vi "Process BD Preview.vi"(9 "Visible Area":T2, 11 "vi ref in":refnum<vi>) -> (1 "BD Preview Center":T1, 3 "BD Preview":picture)   [LabVIEW 2021]
uses:
  <vilib>/Utility/miscctls.llb/LVBoundsTypeDef.ctl
  <vilib>/Utility/miscctls.llb/LVPointTypeDef.ctl
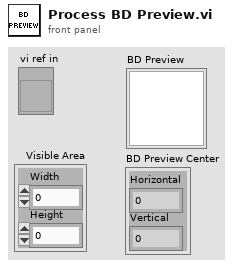
[diagram p1: front panel]
types:
  T1 = typedef "LVPointTypeDef.ctl" = cluster{"Horizontal":i16, "Vertical":i16}
  T2 = typedef "LVBoundsTypeDef.ctl" = cluster{"Width":u32, "Height":u32}
  T3 = typedef "imagedata.ctl" = cluster{"image type":i32, "image depth":i32, "image":u8[], "mask":u8[], "colors":u32[], "Rectangle":cluster{"left":i16, "top":i16, "right":i16, "bottom":i16}}
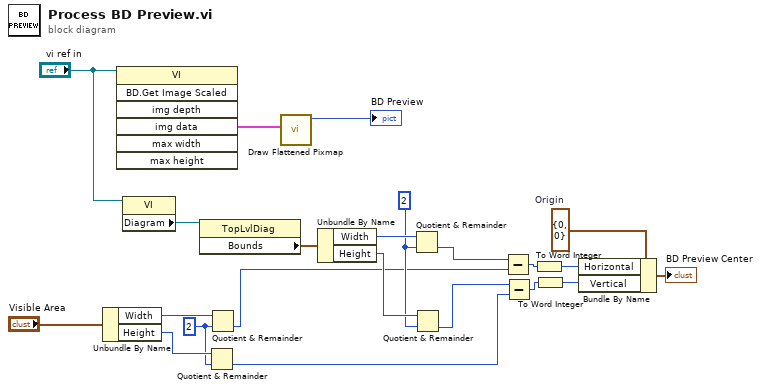
[diagram p0: block diagram]
diagram:
  w2 = T1 {"Horizontal"=0, "Vertical"=0}  # Origin
  w11 = u32 2 ("y")
  w15 = u32 2 ("y")
  n1 = Unbundle By Name("Visible Area") -> ("Width"=w13:u32, "Height"=w12:u32)
  n2 = invoke class="VI" method="BD.Get Image Scaled"(reference="vi ref in") -> ("img data"=w22:T3)  [unwired: 6 in, 6 out]
  n3 = property class="VI"(reference="vi ref in") -> ("Diagram"=w19:refnum<vi>)  [unwired: 1 in, 2 out]
  n4 = property class="TopLvlDiag"(reference=w19) -> ("Bounds"=w18:T2)  [unwired: 1 in, 2 out]
  n5 = Quotient & Remainder(x=w12, y=w11) -> (floor(x/y)=w4:u32)  [unwired: 1 out]
  n6 = Quotient & Remainder(x=w13, y=w11) -> (floor(x/y)=w10:u32)  [unwired: 1 out]
  n7 = call <vilib>:"Draw Flattened Pixmap.vi"("image data"=w22) -> ("new picture"=→"BD Preview":picture)  [unwired: 8 in]
  n8 = Unbundle By Name(w18) -> ("Width"=w17:u32, "Height"=w16:u32)
  n9 = Quotient & Remainder(x=w17, y=w15) -> (floor(x/y)=w5:u32)  [unwired: 1 out]
  n10 = Quotient & Remainder(x=w16, y=w15) -> (floor(x/y)=w3:u32)  [unwired: 1 out]
  n11 = Subtract(x=w5, y=w10) -> (x-y=w8:u32)
  n12 = Subtract(x=w3, y=w4) -> (x-y=w9:u32)
  n13 = To Word Integer(number=w8) -> (16bit integer=w7:i16)
  n14 = To Word Integer(number=w9) -> (16bit integer=w6:i16)
  n15 = Bundle By Name(cluster=w2, "Horizontal"=w7, "Vertical"=w6) -> (→"BD Preview Center":T1)
